vi "Get VI Path.vi"(8 "error in (no error)":errorcluster, 10 "Base path":path, 11 "Selected VI":string) -> (0 "error out":errorcluster, 3 "VI Path":path)   [LabVIEW 2025]
doc: "Returns path of selected VI"
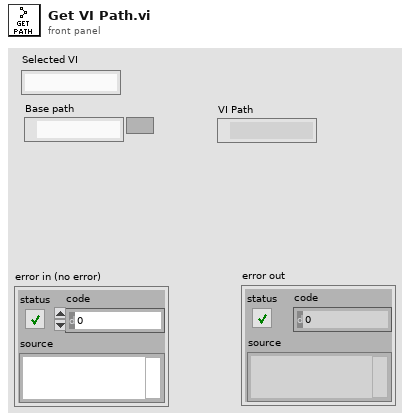
[diagram p1: front panel]
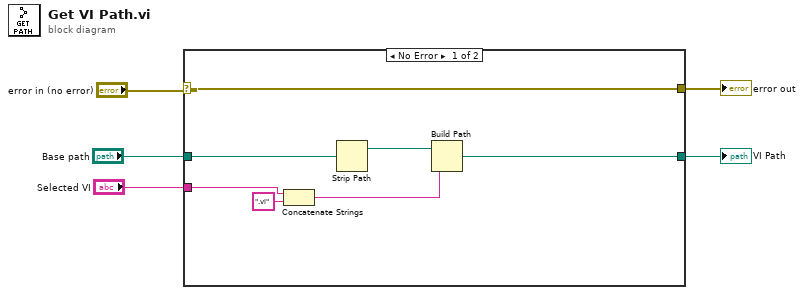
[diagram p0: block diagram]
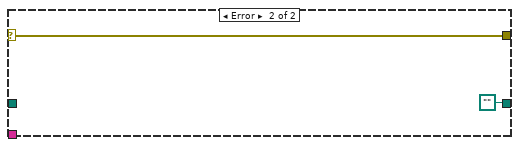
[diagram p2: hidden frame]
diagram:
  n1 = case shown="No Error" "error in (no error)" {
    selector: "error in (no error)" -> [w12 w14]
    tunnel: [w12 w14] -> w4
    tunnel: "Base path" -> [w11 _]
    tunnel: "Selected VI" -> [w9 _]
    tunnel: [w6 path ""] -> w1
    frame No Error {
      n2 = Concatenate Strings(w9, ".vi" ("string")) -> (w7:string)
      n3 = Strip Path(path=w11) -> (stripped path=w10:path)  [unwired: 1 out]
      n4 = Build Path(base path=w10, name or relative path=w7) -> (appended path=w6:path)
    }
    frame Error {
    }
  }
  "VI Path" <- w1
  "error out" <- w4
